vi "util_stop_subs.vi"(8 "error in (no error)":errorcluster, 11 "interface []":T1[](array[typedef])) -> (0 "error out":errorcluster)   [LabVIEW 2015, in "lv-interface-dom-nre.lvlib"]
uses:
  lv-interface-dom-nre.lvlib
  _controls/interface_refnum.ctl
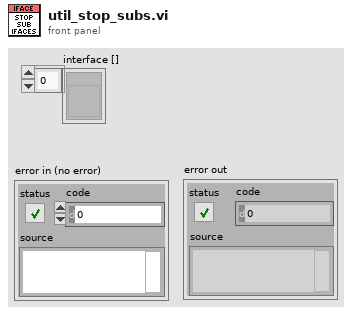
[diagram p1: front panel]
types:
  T1 = typedef "lv-interface-dom-nre.lvlib/interface_refnum.ctl" = refnum<vi>
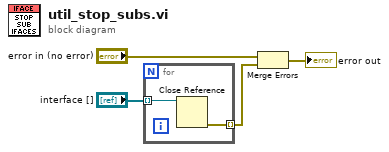
[diagram p0: block diagram]
diagram:
  n1 = for {
    tunnel: "interface []" -> [w6] mode=indexing
    tunnel: [w5] -> w3 mode=indexing
    n2 = Close Reference(reference=w6) -> (error out=w5:errorcluster)  [unwired: 1 in]
  }
  n3 = Merge Errors("error in (no error)", w3) -> (→"error out":errorcluster)
